vi "example_vector_unit_test_1.vi"() -> ()   [LabVIEW 2020]
uses:
  src/vectorstore/abstract_vector_base/abstract_vector_base.lvclass
  src/vectorstore/abstract_vector_base/vector.ctl
  src/models/llm_openai_embedding/llm_openai_embedding.lvclass
  D:/petwork/labview-llm-libraries/src/models/abstract_llm_base/abstract_llm_base.lvclass
  src/vectorstore/vector_qdrant/vector_qdrant.lvclass
  D:/petwork/labview-llm-libraries/src/vectorstore/abstract_vector_base/abstract_vector_base.lvclass
  src/models/message_text/message_text.lvclass
  D:/petwork/labview-llm-libraries/src/models/abstract_message_base/abstract_message_base.lvclass
  src/models/message_vectors/message_vectors.lvclass
  src/models/message_text/create_text_message.vi
  src/models/llm_openai_embedding/Instantiate_llm_openai_embed.vi
  src/models/message_text/get_text_message_value.vi
  src/models/message_vectors/get_vector_message_value.vi
  src/models/abstract_llm_embedding/abstract_llm_embedding.lvclass
  D:/petwork/labview-llm-libraries/src/models/message_text/message_text.lvclass
  D:/petwork/labview-llm-libraries/src/models/message_vectors/message_vectors.lvclass
panel:
  in  "K size":u32=3
  out "Search Results":string[](array[string])
  in  "Search Query":string="Yellow Fruit"
  in  "Database":string[](array[string])=["Apple", "USD", "Mango", "Titanic", "Himalayas", "Papaya", "Barrak Obama", "Drangon Fruit", "Cocnut", "Pacific Ocean", "Banana", "Carrot", "Biscut", "Pokemon", "Cherry", "Mothers day"]
  out "error out":errorcluster
  in  "collection_name":string="my_collection"
  in  "Vector Selector":enum32{"qdrant", "weviate"}(tab)
  in  "host_url":string="http://localhost:6333/"
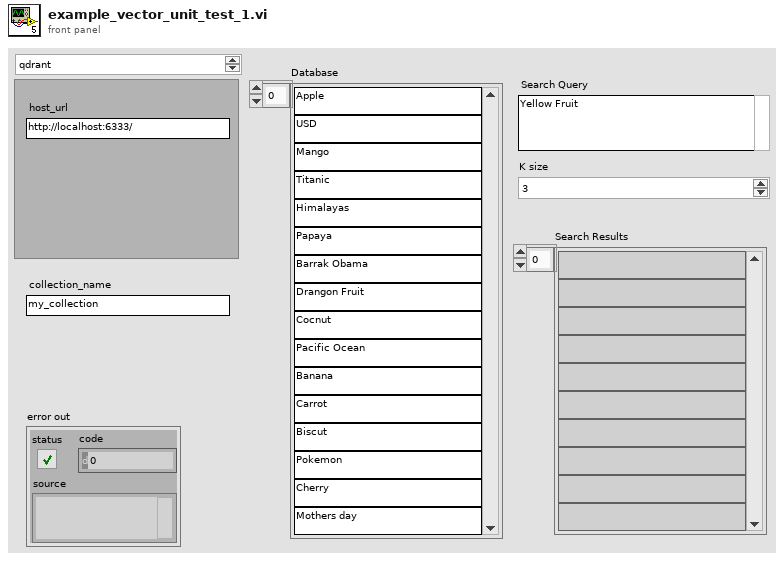
[diagram p1: front panel]
types:
  T1 = typedef "abstract_vector_base.lvclass/vector.ctl" = cluster{"id":string, "vector":dbl[], "text":string, "metadata":cluster{"key":string, "value":string}[]}
  T2 = typedef "message_vectors.lvclass/embedding.ctl" = cluster{"index":u32, "Vectors":dbl[]}
  T3 = typedef "abstract_vector_base.lvclass/search result.ctl" = cluster{"score":dbl, "vector":T1}
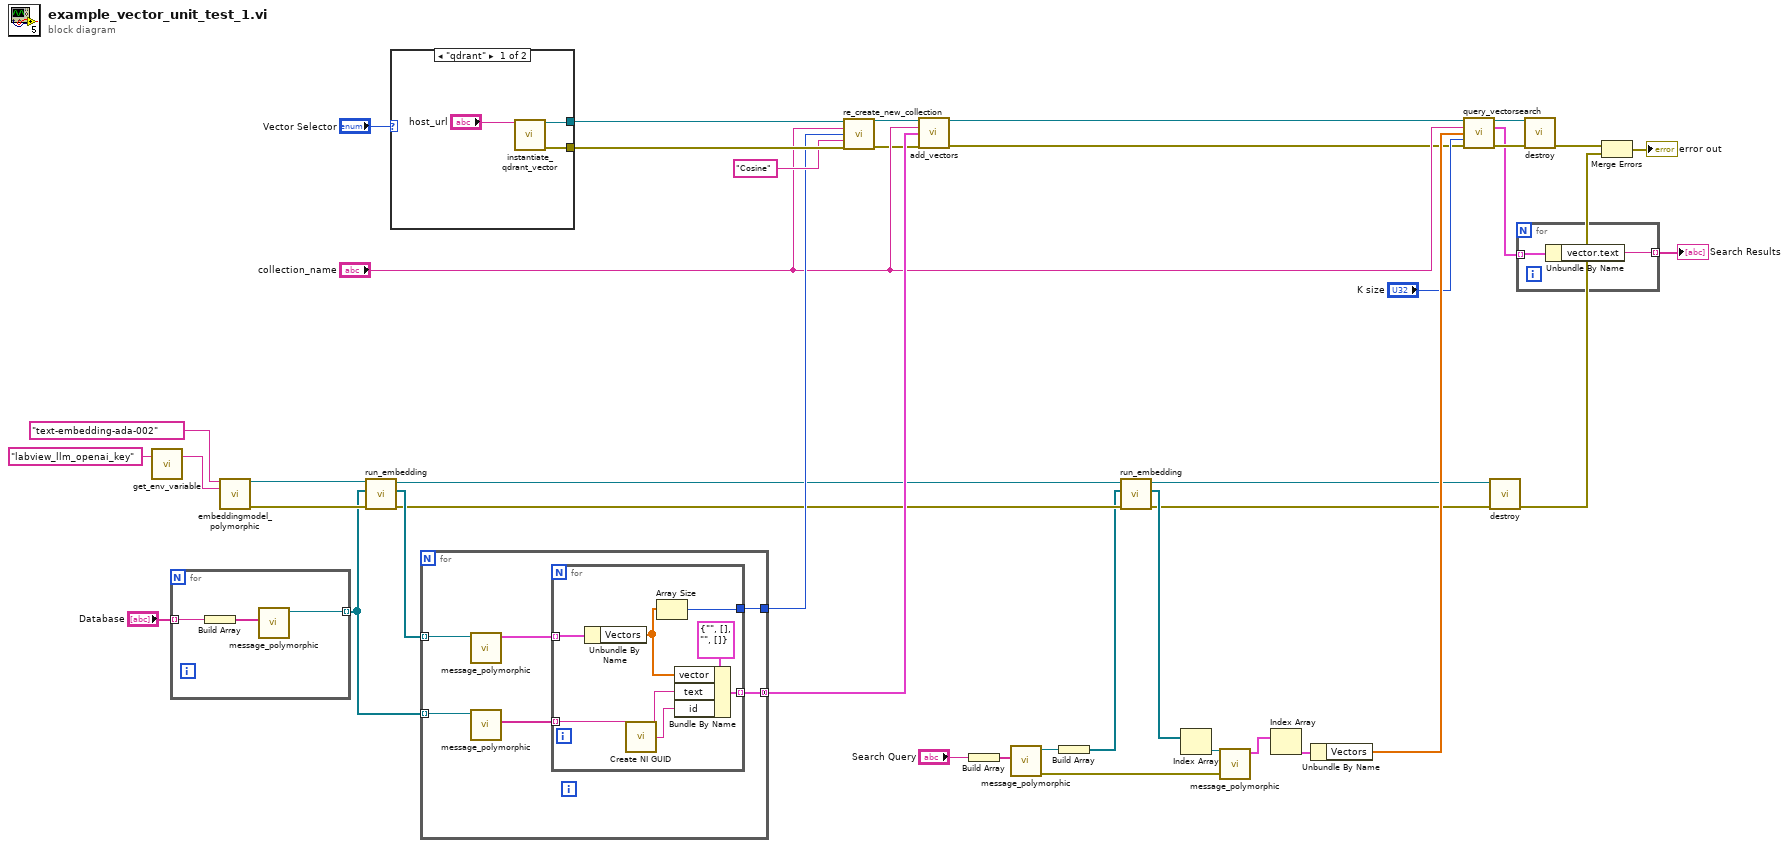
[diagram p0: block diagram]
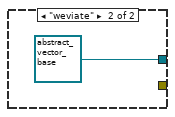
[diagram p2: hidden frame]
diagram:
  n1 = call "get_env_variable.vi"("Environment Variable Name"="labview_llm_openai_key") -> ("Value"=w32:string)  [unwired: 1 in, 1 out]
  n2 = for {
    tunnel: "Database" -> [w44] mode=indexing
    tunnel: [w43] -> w27 mode=indexing
    n3 = Build Array(w44) -> (w42:string[])
    n4 = call-poly "message_polymorphic.vi"("content"=w42) -> ("message_text out"=w43:refnum<class "message_text.lvclass">)  [unwired: 9 in, 1 out]
  }
  n5 = call-poly "embeddingmodel_polymorphic.vi"("model_name"="text-embedding-ada-002", "openai_key"=w32) -> ("llm_openai_embedding out"=w34:refnum<class "llm_openai_embedding.lvclass">, "error out"=w35:errorcluster)  [unwired: 12 in]
  n6 = call "run_embedding.vi"("error in (no error)"=w35, "Messages"=w27, "abstract_llm_embedding in"=w34) -> ("error out"=w18:errorcluster, "Response"=w36:refnum<class "message_vectors.lvclass">[], "abstract_llm_embedding out"=w19:refnum<class "llm_openai_embedding.lvclass">)  [unwired: 6 in]
  n7 = case shown="\"qdrant\"" "Vector Selector" {
    tunnel: [w47 refnum<class "abstract_vector_base.lvclass"> refnum ("abstract_vector_base.lvclass")] -> w39
    tunnel: [w45 _] -> w38
    frame "qdrant" {
      n8 = call "instantiate_qdrant_vector.vi"("host_url"="host_url") -> ("vector_qdrant out"=w47:refnum<class "vector_qdrant.lvclass">, "error out"=w45:errorcluster)  [unwired: 13 in]
    }
    frame "weviate" {
    }
  }
  n9 = for {
    tunnel: w36 -> [w54] mode=indexing
    tunnel: w27 -> [w53] mode=indexing
    tunnel: [w50] -> w25 mode=concatenating
    tunnel: [w49] -> w26
    n10 = call-poly "message_polymorphic.vi"("message_vectors in"=w54) -> ("embedding_data"=w52:T2[])  [unwired: 9 in, 1 out]
    n11 = call-poly "message_polymorphic.vi"("abstract_message_base.lvclass"=w53) -> ("content"=w51:string[])  [unwired: 8 in, 2 out]
    n12 = for {
      tunnel: w52 -> [w60] mode=indexing
      tunnel: w51 -> [w59] mode=indexing
      tunnel: [w58] -> w50 mode=indexing
      tunnel: [w55] -> w49
      n13 = Unbundle By Name(w60) -> ("Vectors"=w57:dbl[])
      n14 = call <vilib>:"Create NI GUID.vi"() -> ("NI GUID"=w56:string)
      n15 = Array Size(array=w57) -> (size(s)=w55:i32)
      n16 = Bundle By Name(cluster=T1 {"id"="", "vector"=[], "text"="", "metadata"=[]} ("vector"), "vector"=w57, "text"=w59, "id"=w56) -> (w58:T1)
    }
  }
  n17 = call-dynamic "re_create_new_collection.vi"("abstract_vector_base in"=w39, "collection_name"="collection_name", "vector_size"=w26, "distance"="Cosine", "error in (no error)"=w38) -> ("abstract_vector_base out"=w2:refnum<class "abstract_vector_base.lvclass">, "error out"=w3:errorcluster)  [unwired: 9 in]
  n18 = call-dynamic "add_vectors.vi"("abstract_vector_base in"=w2, "colection_name"="collection_name", "vectors"=w25, "error in (no error)"=w3) -> ("abstract_vector_base out"=w5:refnum<class "abstract_vector_base.lvclass">, "error out"=w1:errorcluster)  [unwired: 10 in]
  n19 = Build Array("Search Query") -> (w21:string[])
  n20 = call-poly "message_polymorphic.vi"("content"=w21) -> ("error out"=w14:errorcluster, "message_text out"=w20:refnum<class "message_text.lvclass">)  [unwired: 9 in]
  n21 = Build Array(w20) -> (w17:refnum<class "message_text.lvclass">[])
  n22 = call "run_embedding.vi"("error in (no error)"=w18, "Messages"=w17, "abstract_llm_embedding in"=w19) -> ("error out"=w9:errorcluster, "Response"=w16:refnum<class "message_vectors.lvclass">[], "abstract_llm_embedding out"=w8:refnum<class "llm_openai_embedding.lvclass">)  [unwired: 6 in]
  n23 = Index Array(array=w16) -> (element=w15:refnum<class "message_vectors.lvclass">)  [unwired: 1 in]
  n24 = call-poly "message_polymorphic.vi"("error in (no error)"=w14, "message_vectors in"=w15) -> ("embedding_data"=w13:T2[])  [unwired: 8 in, 1 out]
  n25 = Index Array(array=w13) -> (element=w12:T2)  [unwired: 1 in]
  n26 = Unbundle By Name(w12) -> ("Vectors"=w11:dbl[])
  n27 = call-dynamic "query_vectorsearch.vi"("abstract_vector_base in"=w5, "collection_name"="collection_name", "vector"=w11, "limit"="K size", "error in (no error)"=w1) -> ("abstract_vector_base out"=w24:refnum<class "abstract_vector_base.lvclass">, "results"=w7:T3[], "error out"=w23:errorcluster)  [unwired: 8 in]
  n28 = call-dynamic "destroy.vi"("error in (no error)"=w9, "llm_openai_embedding in"=w8) -> ("error out"=w28:errorcluster)  [unwired: 8 in, 1 out]
  n29 = for {
    tunnel: w7 -> [w63] mode=indexing
    tunnel: [w62] -> w6 mode=indexing
    n30 = Unbundle By Name(w63) -> ("vector.text"=w62:string)
  }
  "Search Results" <- w6
  n31 = call-dynamic "destroy.vi"("abstract_vector_base in"=w24, "error in (no error)"=w23) -> ("error out"=w40:errorcluster)  [unwired: 12 in, 1 out]
  n32 = Merge Errors(w40, w28) -> (→"error out":errorcluster)
